vi "Read Fluence Infos.vi"(8 "error in (no error)":errorcluster, 11 "Analyze Results Fluence in":refnum<class "Analyze Results Fluence.lvclass">) -> (0 "error out":errorcluster, 2 "Fluence Infos":T1[](array[typedef]), 3 "Analyze Results Fluence out":refnum<class "Analyze Results Fluence.lvclass">)   [LabVIEW 2014, in "Analyze Results Fluence.lvclass"]
uses:
  Analyze Results Fluence.lvclass
  Analyze Classes/Analyze Fluence/Fluence Info.ctl
  Analyze Results Fluence.lvclass/Analyze Results Fluence.ctl
  Analyze Classes/Analyze Fluence/Analyze Fluence.lvclass
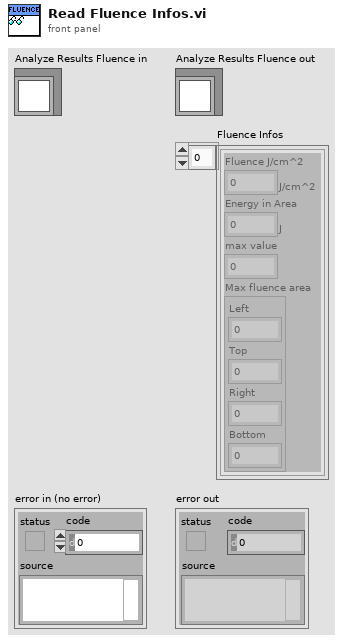
[diagram p1: front panel]
types:
  T1 = typedef "Analyze.lvlib/Analyze Fluence.lvclass/Fluence Info.ctl" = cluster{"Fluence J/cm^2":dbl[unit], "Energy in Area":dbl[unit], "max value":i64, "Max fluence area":cluster{"Left":i32, "Top":i32, "Right":i32, "Bottom":i32}}
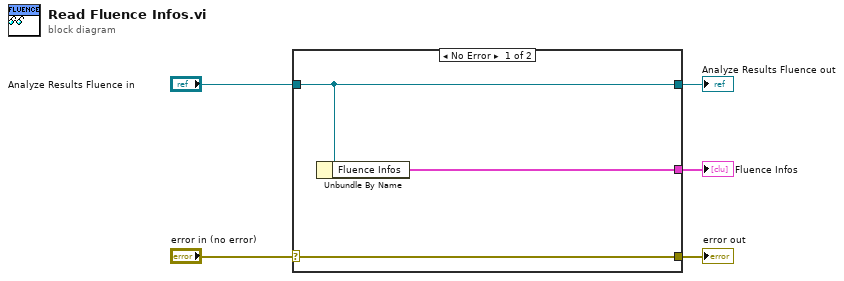
[diagram p0: block diagram]
diagram:
  n1 = case shown="No Error" "error in (no error)" {
    selector: "error in (no error)" -> [w8 w9]
    tunnel: [w8 w9] -> w4
    tunnel: [w7 w10] -> w2
    tunnel: "Analyze Results Fluence in" -> [w7 w10]
    tunnel: [w6 _] -> w1
    frame No Error {
      n2 = Unbundle By Name(w7) -> ("Fluence Infos"=w6:T1[])
    }
    frame Error {
    }
  }
  "error out" <- w4
  "Analyze Results Fluence out" <- w2
  "Fluence Infos" <- w1
